vi "Trigger Reading.vi"(2 "Old Trigger Value":dbl format="%.2f", 3 "Current Values":dbl[](array[numeric]) format="%.2e", 4 "Trigger Column":i32, 5 "Æ Trigger Value":dbl format="%.2f") -> (0 "New Trigger Value":dbl format="%.2e", 1 "Wait":bool)   [LabVIEW 2025]
doc: "Decides if the inputs have changed by an amount greater than delta so that a reading is triggered (saved).\nScott Hannahs, FBNML, Jan 1992\nAuthor: Scott Hannahs <sth@magnet.fsu.edu>\n\nThis software is licensed for use under the “MIT License\"\nCopyright (c) 2025 Scott Hannahs, sth@sth@magnet.sthnet.net\n\nPermission is hereby granted, free of charge, to any person obtaining a copy of this software and associated documentation files (the \"Software\"), to deal in the Software without restriction, including without limitation the rights to use, copy, modify, merge, publish, distribute, sublicense, and/or sell copies of the Software, and to permit persons to whom the Software is furnished to do so, subject to the following conditions: The above copyright notice and this permission notice shall be included in all copies or substantial portions of the Software.\n\nTHE SOFTWARE IS PROVIDED \"AS IS\", WITHOUT WARRANTY OF ANY KIND, EXPRESS OR IMPLIED, INCLUDING BUT NOT LIMITED TO THE WARRANTIES OF MERCHANTABILITY, FITNESS FOR A PARTICULAR PURPOSE AND NONINFRINGEMENT. IN NO EVENT SHALL THE AUTHORS OR COPYRIGHT HOLDERS BE LIABLE FOR ANY CLAIM, DAMAGES OR OTHER LIABILITY, WHETHER IN AN ACTION OF CONTRACT, TORT OR OTHERWISE, ARISING FROM, OUT OF OR IN CONNECTION WITH THE SOFTWARE OR THE USE OR OTHER DEALINGS IN THE SOFTWARE."
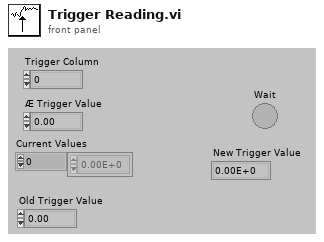
[diagram p1: front panel]
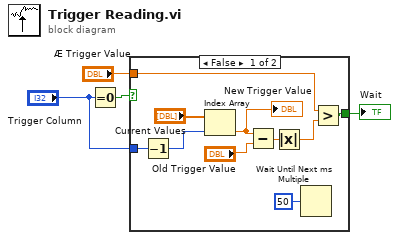
[diagram p0: block diagram]
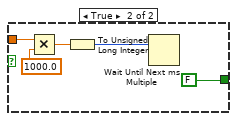
[diagram p2: hidden frame]
diagram:
  n1 = Equal To 0?(x="Trigger Column") -> (x = 0?=w4:bool)
  n2 = case shown="False" w4 {
    tunnel: [w8 FALSE] -> w1
    tunnel: "Æ Trigger Value" -> [w11 w17]
    tunnel: "Trigger Column" -> [w13 _]
    frame False {
      n3 = Decrement(x=w13) -> (x-1=w6:i32)
      n4 = Index Array(array="Current Values", index=w6) -> (element=w7:dbl)
      "New Trigger Value" <- w7
      n5 = Subtract(x=w7, y="Old Trigger Value") -> (x-y=w10:dbl)
      n6 = Absolute Value(x=w10) -> (abs(x)=w9:dbl)
      n7 = Wait Until Next ms Multiple(millisecond multiple=u32 50) -> ()  [unwired: 1 out]
      n8 = Greater?(x=w11, y=w9) -> (0:w8:bool)
    }
    frame True {
      n9 = Multiply(x=w17, y=1000.0) -> (x*y=w16:dbl)
      n10 = To Unsigned Long Integer(number=w16) -> (unsigned 32bit integer=w15:u32)
      n11 = Wait Until Next ms Multiple(millisecond multiple=w15) -> ()  [unwired: 1 out]
    }
  }
  "Wait" <- w1
